vi "Load Module--non-reentrant.vi"(8 "error in":errorcluster, 11 "Config Section":string) -> (0 "error out":errorcluster, 2 "Broadcast Events":T1, 3 "Module ID (dup)":i32)   [LabVIEW 2014, in "DB_CONNECTOR.lvlib"]
uses:
  DB_CONNECTOR.lvlib
  Broadcast Events--cluster.ctl
  Did Init Argument--cluster.ctl
  Status Updated Argument--cluster.ctl
  Error Reported Argument--cluster.ctl
  Stop Argument--cluster.ctl
  Get Module Execution Status Argument--cluster.ctl
  Fast Query Reply Argument--cluster.ctl
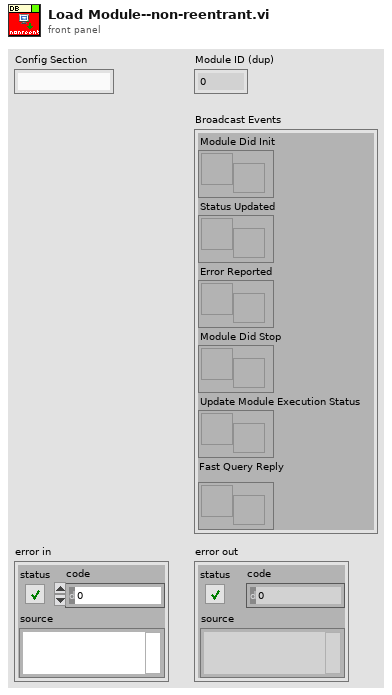
[diagram p1: front panel]
types:
  T1 = typedef "DB_CONNECTOR.lvlib/Broadcast Events--cluster.ctl" = cluster{"Module Did Init":refnum<user-event>, "Status Updated":refnum<user-event>, "Error Reported":refnum<user-event>, "Module Did Stop":refnum<user-event>, "Update Module Execution Status":refnum<user-event>, "Fast Query Reply":refnum<user-event>}
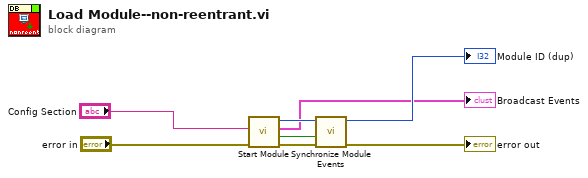
[diagram p0: block diagram]
diagram:
  n1 = call "Start Module.vi"("error in (no error)"="error in", "Config Section"="Config Section") -> ("error out"=w7:errorcluster, "Wait for Event Sync?"=w8:bool, "DB_CONNECTOR Broadcast Events"=→"Broadcast Events":T1, "Module ID"=w6:i32)  [unwired: 6 in]
  n2 = call "Synchronize Module Events.vi"("error in (no error)"=w7, "Wait for Event Sync?"=w8, "Module ID"=w6) -> ("error out"=→"error out":errorcluster, "Module ID (dup)"=→"Module ID (dup)":i32)  [unwired: 7 in]
